vi "Untitled 1.vi"() -> ()   [LabVIEW 2010]
uses:
  <vilib>/NXT/Block Support/NXT_InputPort.ctl
  <vilib>/NXT/Subs/MotorOutput.ctl
  <vilib>/NXT/Dual Mode Library/Sensors/Sonar_cm.vi
  <vilib>/NXT/Dual Mode Library/Motors/MotorReverse.vi
  <vilib>/NXT/Dual Mode Library/Waits/Wait_Rotation.vi
  <vilib>/NXT/Dual Mode Library/Motors/MotorOn.vi
  <vilib>/NXT/Dual Mode Library/Waits/Wait_Num.vi
  <vilib>/NXT/Dual Mode Library/Waits/Wait_Brightness.vi
panel:
  in  "stop":bool
  in  "빛센서 포트":T1=2 caption="Port (Port 3)" items=["Port 1", "Port 2", "Port 3", "Port 4"]
  in  "Power (75)":i32=75
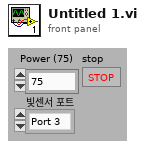
[diagram p1: front panel]
types:
  T1 = typedef "NXT_InputPort.ctl" = u8
  T2 = typedef "MotorOutput.ctl" = u8
  T3 = typedef "LVHSConnector.ctl" = cluster{"error":errorcluster, "address":string, "NXT #":i32, "Show Error":bool, "Connection":u16}
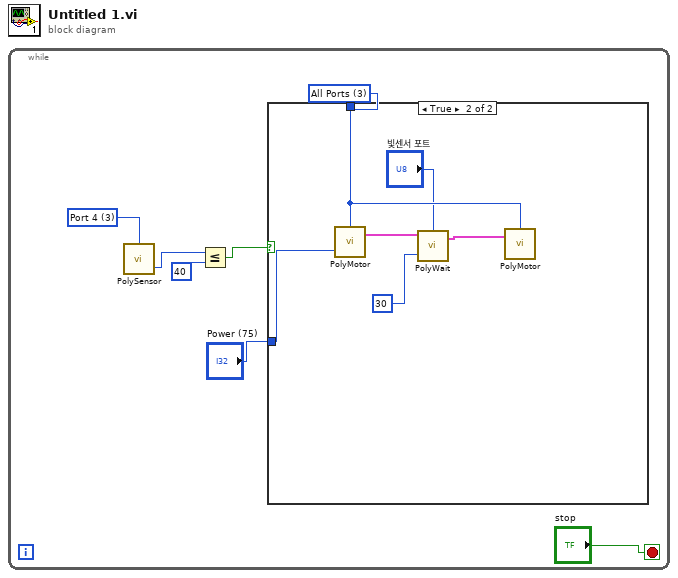
[diagram p0: block diagram]
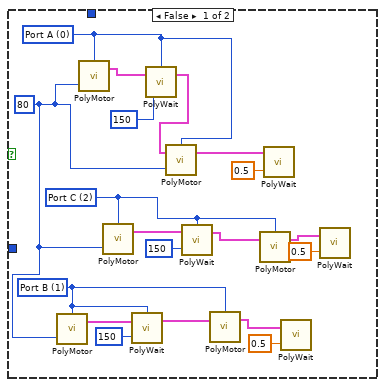
[diagram p2: hidden frame]
diagram:
  n1 = while {
    stop <- "stop" stop-if-true
    w3 = T2 3 items=["Port A", "Port B", "Port C", "All Ports"] ("Output Port (All Ports)")
    w7 = T1 3 items=["Port 1", "Port 2", "Port 3", "Port 4"] ("Port (Port 4)")
    n2 = call-poly <vilib>:"PolySensor.vi"("Port (Port 4)"=w7) -> ("Distance (cm)"=w6:i16)  [unwired: 2 in, 1 out]
    n3 = Less Or Equal?(x=w6, y=i16 40) -> (x <= y?=w4:bool)
    n4 = case shown="True" w4 {
      tunnel: w3 -> [_ w30]
      tunnel: "Power (75)" -> [_ w32]
      frame False {
        w8 = 80 ("Power (75)")
        w16 = T2 1 items=["Port A", "Port B", "Port C", "All Ports"] ("Output Port (All Ports)")
        w21 = T2 2 items=["Port A", "Port B", "Port C", "All Ports"] ("Output Port (All Ports)")
        w26 = T2 0 items=["Port A", "Port B", "Port C", "All Ports"] ("Output Port (All Ports)")
        n5 = call-poly <vilib>:"PolyMotor.vi"("Power (75)"=w8, "Output Port (All Ports)"=w16) -> ("NXT"=w15:T3)  [unwired: 2 in]
        n6 = call-poly <vilib>:"PolyMotor.vi"("Power (75)"=w8, "Output Port (All Ports)"=w26) -> ("NXT"=w25:T3)  [unwired: 2 in]
        n7 = call-poly <vilib>:"PolyMotor.vi"("Power (75)"=w8, "Output Port (All Ports)"=w21) -> ("NXT"=w20:T3)  [unwired: 2 in]
        n8 = call-poly <vilib>:"PolyWait.vi"("Position Change (180)"=150, "NXT"=w15, "Port (Port A)"=w16) -> ("NXT"=w14:T3)  [unwired: 1 in]
        n9 = call-poly <vilib>:"PolyWait.vi"("Position Change (180)"=150, "NXT"=w25, "Port (Port A)"=w26) -> ("NXT"=w24:T3)  [unwired: 1 in]
        n10 = call-poly <vilib>:"PolyMotor.vi"("Power (75)"=w8, "NXT"=w24, "Output Port (All Ports)"=w26) -> ("NXT"=w23:T3)  [unwired: 1 in]
        n11 = call-poly <vilib>:"PolyWait.vi"("Position Change (180)"=150, "NXT"=w20, "Port (Port A)"=w21) -> ("NXT"=w19:T3)  [unwired: 1 in]
        n12 = call-poly <vilib>:"PolyMotor.vi"("NXT"=w14, "Output Port (All Ports)"=w16) -> ("NXT"=w13:T3)  [unwired: 2 in]
        n13 = call-poly <vilib>:"PolyMotor.vi"("NXT"=w19, "Output Port (All Ports)"=w21) -> ("NXT"=w18:T3)  [unwired: 2 in]
        n14 = call-poly <vilib>:"PolyWait.vi"("Time (1 sec)"=sgl 0.5 ("Time (sec)"), "NXT"=w23) -> ()  [unwired: 2 in, 1 out]
        n15 = call-poly <vilib>:"PolyWait.vi"("Time (1 sec)"=sgl 0.5 ("Time (sec)"), "NXT"=w13) -> ()  [unwired: 2 in, 1 out]
        n16 = call-poly <vilib>:"PolyWait.vi"("Time (1 sec)"=sgl 0.5 ("Time (sec)"), "NXT"=w18) -> ()  [unwired: 2 in, 1 out]
      }
      frame True {
        n17 = call-poly <vilib>:"PolyMotor.vi"("Power (75)"=w32, "Output Port (All Ports)"=w30) -> ("NXT"=w29:T3)  [unwired: 2 in]
        n18 = call-poly <vilib>:"PolyWait.vi"("Brightness (40)"=u8 30, "NXT"=w29, "Port (Port 3)"="빛센서 포트") -> ("NXT"=w28:T3)  [unwired: 1 in]
        n19 = call-poly <vilib>:"PolyMotor.vi"("NXT"=w28, "Output Port (All Ports)"=w30) -> ()  [unwired: 2 in, 1 out]
      }
    }
  }
